vi "Calculate-Checksum.vi"(9 "Array":u8[](array[numeric]) format="%.0x") -> (0 "Checksum":u16 format="%04x", 1 "Checksum OK?":bool)   [LabVIEW 2017]
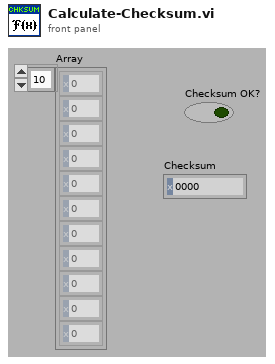
[diagram p1: front panel]
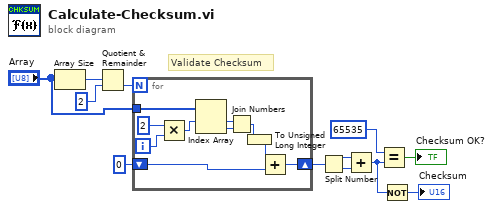
[diagram p0: block diagram]
diagram:
  # "Validate Checksum"
  n1 = Array Size(array="Array") -> (size(s)=w9:i32)
  n2 = Quotient & Remainder(x=w9, y=2) -> (floor(x/y)=w7:i32)  [unwired: 1 out]
  n3 = for {
    N: w7 -> [_]
    tunnel: "Array" -> [w22]
    shift-right: [w17] -> w3
    shift-left: u32 0 ("y") -> [w18]
    i -> [w21]
    n4 = Multiply(x=2, y=w21) -> (x*y=w19:i32)
    n5 = Index Array(array=w22, index #1=w19) -> (element #1=w16:u8, element #2=w15:u8)  [unwired: 1 in]
    n6 = Join Numbers(hi=w16, lo=w15) -> ((hi.lo)=w14:u16)
    n7 = To Unsigned Long Integer(number=w14) -> (unsigned 32bit integer=w13:u32)
    n8 = Add(x=w13, y=w18) -> (x+y=w17:u32)
  }
  n9 = Split Number(x=w3) -> (hi(x)=w12:u16, lo(x)=w2:u16)
  n10 = Add(x=w12, y=w2) -> (x+y=w1:u16)
  n11 = Equal?(x=u16 65535, y=w1) -> (x = y?=→"Checksum OK?":bool)
  n12 = Not(x=w1) -> (.not. x?=→"Checksum":u16)
